vi "Set the Volt Interval According to Range in Autosetup_FP-Scope SP.vi"(7 "PP":dbl) -> (8 "VoltInterval":i32)   [LabVIEW 2012]
doc: "根据自动调整后的range获取voltinterval"
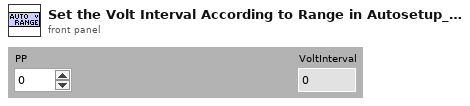
[diagram p1: front panel]
types:
  T1 = typedef "INI Properties_DStr-Scope SP.ctl" = cluster{"Channels":cluster{"String":string, "Value":ext}[], "VoltInterval":cluster{"String":string, "Value":ext}[], "Impedance":cluster{"String":string, "Value":ext}[], "Bandwidth":cluster{"String":string, "Value":ext}[], "TimeInterval":cluster{"String":string, "Value":ext}[], "Type":cluster{"String":string, "Value":ext}[], "Source":cluster{"String":string, "Value":ext}[], "DigiSource":cluster{"String":string, "Value":ext}[], "TrigCpl":cluster{"String":string, "Value":ext}[], "EXTCpl":cluster{"String":string, "Value":ext}[], "Mode":cluster{"String":string, "Value":ext}[], "Event":cluster{"String":string, "Value":ext}[], "Format":cluster{"String":string, "Value":ext}[], "OffsetVisible":bool[], "Offset":dbl[][], "Point":dbl[][], "TrigLev":dbl[][], "Win":dbl[][], "Leve":dbl[][], "ExtLev":dbl[][], "PolaEnable":u8, "RISEnable":u8, "ChanCpl":cluster{"String":string, "Value":ext}[], "TimeValue":dbl[], "VoltValue":dbl[], "ImpedanceValue":dbl[], "BandwidthValue":dbl[]}
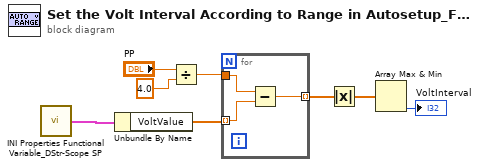
[diagram p0: block diagram]
diagram:
  n1 = call "INI Properties Functional Variable_DStr-Scope SP.vi"() -> ("proper"=w2:T1)  [unwired: 15 in]
  n2 = Unbundle By Name(w2) -> ("VoltValue"=w1:dbl[])
  n3 = Divide(x="PP", y=4.0 ("x")) -> (x/y=w7:dbl)
  n4 = for {
    tunnel: w1 -> [w10] mode=indexing
    tunnel: w7 -> [w11]
    tunnel: [w9] -> w5 mode=indexing
    n5 = Subtract(x=w11, y=w10) -> (x-y=w9:dbl)
  }
  n6 = Absolute Value(x=w5) -> (abs(x)=w4:dbl[])
  n7 = Array Max & Min(array=w4) -> (min index (indices)=→"VoltInterval":i32)  [unwired: 3 out]
